vi "set exit code.vi"(11 "exit code":i32) -> ()   [LabVIEW 2013]
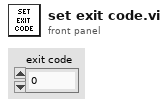
[diagram p1: front panel]
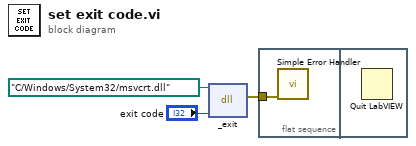
[diagram p0: block diagram]
diagram:
  n1 = dll-call lib="C:/Windows/System32/msvcrt.dll" fn="_exit"(path in=path "C:/Windows/System32/msvcrt.dll", "code"="exit code") -> (error out=w2:errorcluster)  [unwired: 4 in, 1 out]
  n2 = flat-sequence {
    tunnel: w2 -> [w4]
    frame #0 {
      n3 = call <vilib>:"Simple Error Handler.vi"("error in (no error)"=w4) -> ()  [unwired: 4 in, 5 out]
    }
    frame #1 {
      n4 = Quit LabVIEW() -> ()  [unwired: 1 in]
    }
  }
